vi "SUB_GET_DATE.vi"() -> ()   [LabVIEW 2011]
panel:
  out "standard output":string
  out "Photo_location":string
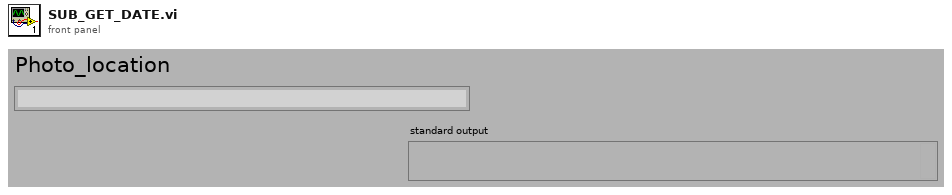
[diagram p1: front panel]
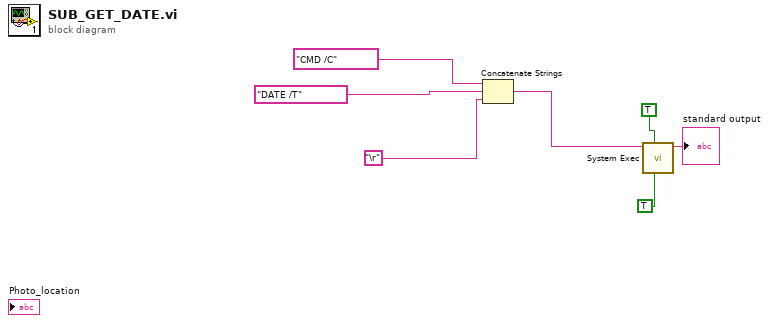
[diagram p0: block diagram]
diagram:
  n1 = Concatenate Strings("CMD /C", "DATE /T", "\r") -> (w5:string)
  n2 = call <vilib>:"System Exec.vi"("run minimized? (F)"=TRUE, "wait until completion? (T)"=TRUE, "command line"=w5) -> ("standard output"=→"standard output":string)  [unwired: 5 in, 3 out]
